vi "Data Viewer.vi"() -> ()   [LabVIEW 2018]
uses:
  <vilib>/drjdpowell/SQLite Library/SQL Connection/Open (path).vi
  <vilib>/drjdpowell/SQLite Library/SQL Connection/Open (string).vi
  <vilib>/AdvancedString/Path To Command Line String.vi
  <vilib>/drjdpowell/SQLite Library/SQL Connection/Execute SQL (1D String).vi
  <vilib>/drjdpowell/SQLite Library/SQL Connection/Execute SQL.vi
  <vilib>/drjdpowell/SQLite Library/SQL Connection/Connection.lvclass
  <vilib>/drjdpowell/SQLite Library/SQLite.lvlib
panel:
  in  "stop":bool
  in  "Tab Control":enum32{"Daily", "Search"}(tab)
  in  "OK":bool caption="Start"
  in  "Time Stamp":timestamp format="%<%Y/%m/%d>T"
  out "Day Result":string[][](table) caption="Result Set (from first statement with results)"
  in  "dbPath":path=path "D:/Valeo/Micriphone Test/UI/data.s3db"
  # "Under Construction"
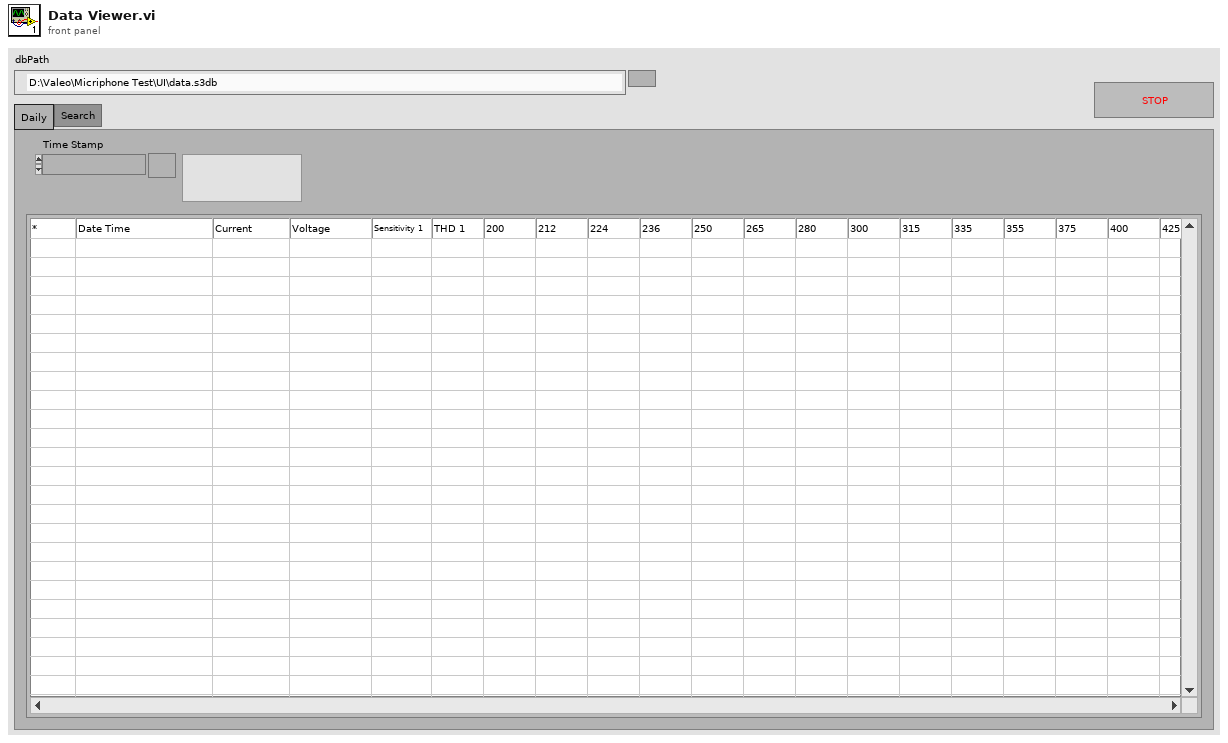
[diagram p1: front panel]
types:
  T1 = enum16{"New or existing", "Existing", "Read only"}
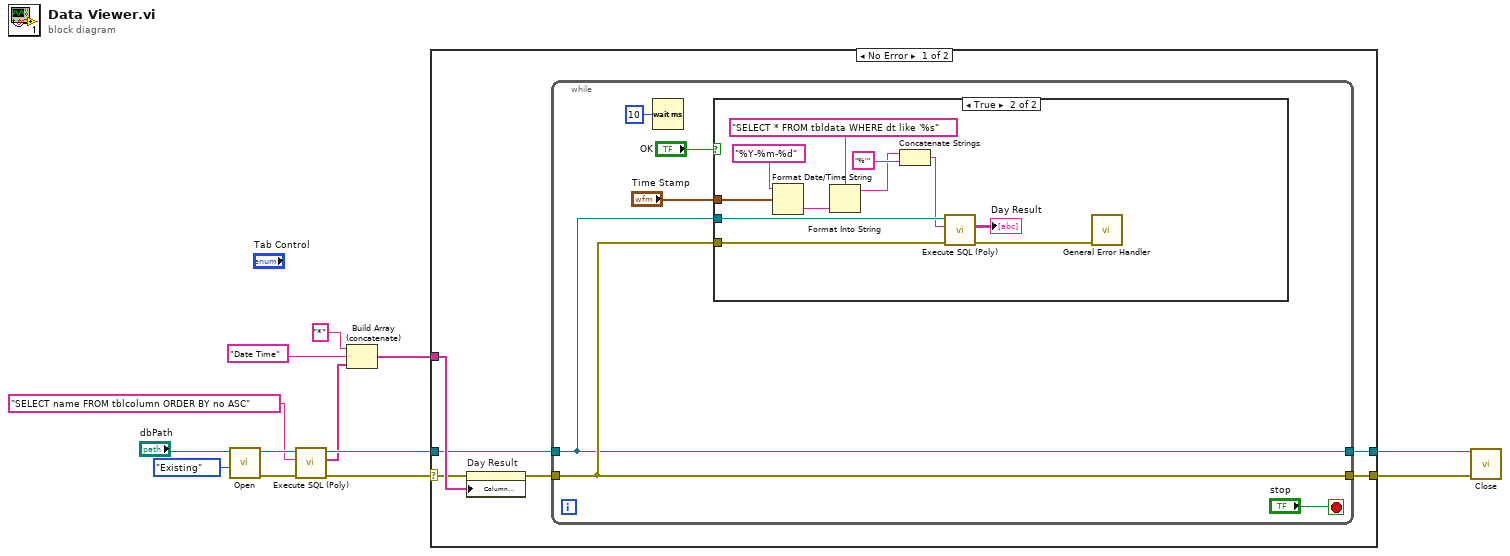
[diagram p0: block diagram]
diagram:
  n1 = call-poly <vilib>:"Open.vi"("File Option"=T1."Existing", "db file"="dbPath") -> ("error out"=w8:errorcluster, "SQLite Connection"=w9:refnum<class "Connection.lvclass">)  [unwired: 8 in]
  n2 = call-poly <vilib>:"Execute SQL (Poly).vi"("error in (no error)"=w8, "SQL"="SELECT name FROM tblcolumn ORDER BY no ASC", "SQLite Connection in"=w9) -> ("error out"=w6:errorcluster, "Result Set"=w2:string[], "SQLite Connection"=w5:refnum<class "Connection.lvclass">)  [unwired: 5 in, 1 out]
  n3 = Build Array (concatenate)("*", "Date Time", w2) -> (w1:string[])
  n4 = case shown="No Error" w6 {
    selector: w6 -> [w16 w38]
    tunnel: w5 -> [w14 w37]
    tunnel: [w19 w38] -> w11
    tunnel: [w18 w37] -> w10
    tunnel: w1 -> [w17 _]
    frame No Error {
      n5 = property on="Day Result" class="Tbl (strict)"(error in=w16, "Column Headers[]"=w17) -> (error out=w15:errorcluster)  [unwired: 1 in, 1 out]
      n6 = while {
        tunnel: w15 -> [w21]
        tunnel: w14 -> [w20]
        tunnel: [w21] -> w19
        tunnel: [w20] -> w18
        stop <- "stop" stop-if-true
        n7 = Wait (ms)(milliseconds to wait=u32 10) -> ()  [unwired: 1 out]
        n8 = case shown="True" "OK" {
          tunnel: "Time Stamp" -> [_ w35]
          tunnel: w21 -> [_ w33]
          tunnel: w20 -> [_ w32]
          frame False {
          }
          frame True {
            n9 = Format Date/Time String(time format string (%c)="%Y-%m-%d", seconds (now)=w35) -> (date/time string=w34:string)  [unwired: 1 in]
            n10 = Format Into String(format string="SELECT * FROM tbldata WHERE dt like '%s", w34) -> (resulting string=w27:string)  [unwired: 2 in, 1 out]
            n11 = Concatenate Strings(w27, "%'") -> (w26:string)
            n12 = call-poly <vilib>:"Execute SQL (Poly).vi"("error in (no error)"=w33, "SQL"=w26, "SQLite Connection in"=w32) -> ("error out"=w30:errorcluster, "Result Set"=→"Day Result":string[][])  [unwired: 5 in, 2 out]
            n13 = call <vilib>:"General Error Handler.vi"("error in (no error)"=w30) -> ()  [unwired: 10 in, 5 out]
          }
        }
      }
    }
    frame Error {
    }
  }
  n14 = call-dynamic "Close.vi"("error in (no error)"=w11, "SQLite Connection in"=w10) -> ()  [unwired: 9 in, 1 out]
